vi "Uncertainty Selector.vi"(5 "Default du":dbl, 7 "Default dL":dbl, 8 "df":dbl, 9 "dL":dbl, 10 "du":dbl, 11 "Default df":dbl) -> (0 "df out":dbl, 1 "dL out":dbl, 2 "du out":dbl)   [LabVIEW 2015]
panel:
  # "Inputs"
  # "Outputs"
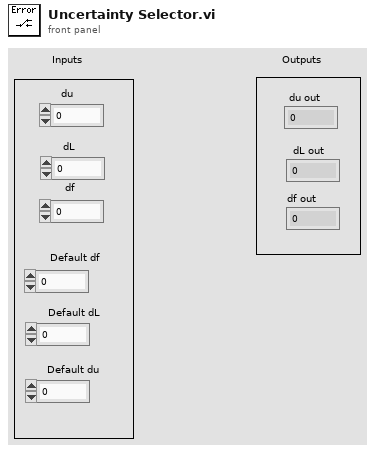
[diagram p1: front panel]
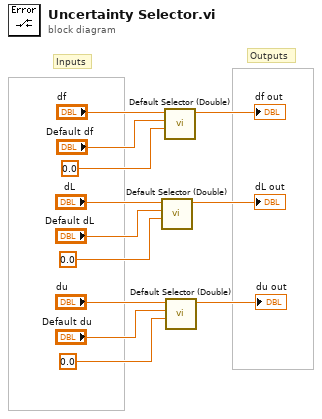
[diagram p0: block diagram]
diagram:
  # "Outputs"
  # "Inputs"
  n1 = call "Default Selector (Double).vi"("Null Input"=0.0, "Default Value"="Default dL", "Input Value"="dL") -> ("Output Value"=→"dL out":dbl)  [unwired: 8 in]
  n2 = call "Default Selector (Double).vi"("Null Input"=0.0, "Default Value"="Default df", "Input Value"="df") -> ("Output Value"=→"df out":dbl)  [unwired: 8 in]
  n3 = call "Default Selector (Double).vi"("Null Input"=0.0, "Default Value"="Default du", "Input Value"="du") -> ("Output Value"=→"du out":dbl)  [unwired: 8 in]
